vi "Player Name.vi"(11 "MyTeam in":refnum<class "MyTeam.lvclass">) -> (2 "Player Name":string)   [LabVIEW 2020, in "SquareTeam.lvlib" / "MyTeam.lvclass"]
uses:
  MyTeam.lvclass
  MyTeam.lvclass/MyTeam.ctl
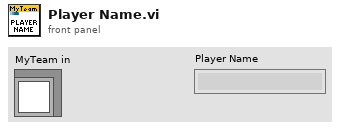
[diagram p1: front panel]
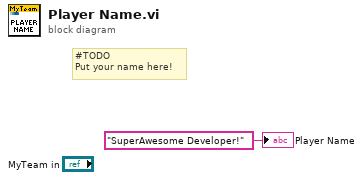
[diagram p0: block diagram]
diagram:
  # "#TODO\nPut your name here!"
  "Player Name" <- "SuperAwesome Developer!" ("Player Name")
